vi "Relay test.vi"() -> ()   [LabVIEW 2021]
uses:
  enums/main_prog_state.ctl
  enums/init_state.ctl
  Master CR.lvclass
  Param/TCP Param/TCP Param.lvclass
  D:/my_projects/projects/Algorithms/Labview/21/Master CR/Param/Param.lvclass
  Master CR.lvclass/Master CR.ctl
  Param/Param.lvclass/Param.ctl
  Param/TCP Param/TCP Param.lvclass/TCP Param.ctl
  <vilib>/Platform/TimedLoop/XDataNode/timing_clust.ctl
  <vilib>/Platform/TimedLoop/XDataNode/nitl_modes.ctl
  <vilib>/Platform/TimedLoop/XDataNode/wakeup.ctl
  enums/close_state.ctl
  Data/Data Model/Read Data Model.vi
  <vilib>/Utility/config.llb/Read Key (String).vi
  <vilib>/Utility/config.llb/Write Key (String).vi
  <vilib>/Platform/TimedLoop/XDataNode/XDataNode.xnode
  Modbus_v121c/Data Model/Device Data Model.lvclass
  <vilib>/Platform/TimedLoop/XDataNode/XDNodeRunTimeDep.lvlib
  enums/Param_MB test.lvlib
  Param/Param.lvclass
  <vilib>/Utility/config.llb/NI_LVConfig.lvlib
panel:
  out "N2":u64
  out "N1":u64
  in  "Write":bool
  in  "Read":bool
  out "connects":bool[](array[boolean])
  out "DI":bool[](array[boolean])
  in  "DO":bool[](array[boolean])
  in  "AOint":u16[](array[numeric])
  out "comm error":errorcluster
  out "initialise error":errorcluster
  in  "EP_on":bool
  in  "tick":i64=250 caption="Время цикла основной программы" min=5 max=1000 step=1
  in  "stop":bool
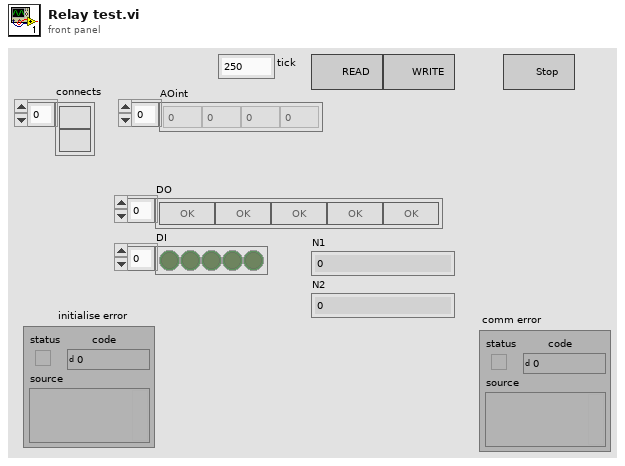
[diagram p1: front panel]
types:
  T1 = cluster{"conn_timeout":i32, "reconn_timeout":i32, "N attempt max":i32, "t_reset_TTL":i32, "write_timeout":i32, "read_timeout":i32, "period":i32}[]
  T2 = cluster{"Remote IP Address":string, "Remote Port":u16}[]
  T3 = typedef "Param_MB test.lvlib/init_state.ctl" = enum16{"Init Data", "Init TMPs", "Init system DB", "Init data DB", "Read Enums", "Init arrays", "Init KFM", "Init Param", "Init AI param", "Init DI param", "Init AO param", "Init DO param", "Init ALR param", "Init save progs", "Read OPC param", "Init Shared Variables", "Init regulators", "Init heaters", "Init Y defs", "Exit"}
  T4 = typedef "Param_MB test.lvlib/main_prog_state.ctl" = enum16{"Read_AI_Param", "Read_DI_Param", "Read_AO_Param", "Read_DO_Param", "Read_ALR_ON_OFF", "Read_ALR_Param", "Read_Param", "Read_REG_Param", "Timers", "AI", "DI", "SendAItoScada", "SendDItoScada", "Alarms", "SendAItoDB", "SendDItoDB", "SendALRtoDB", "Messages", "Controls", "Control HT1", "QN_control", "QN", "QN_state", "Control EB3", "Outputs", "Exit"}
  T5 = cluster{"KFM":string[], "PAR":string[], "AI":string[], "DI":string[], "DI_fast":string[], "AO":string[], "Regs":string[], "DO":string[], "ALR":string[], "System":string[]}
  T6 = typedef "NI_LVConfig.lvlib/Config Data RefNum.ctl" = refnum<k1>
  T7 = cluster{"Enums":cluster{"KFM":string[], "PAR":string[], "AI":string[], "DI":string[], "DI_fast":string[], "AO":string[], "Regs":string[], "DO":string[], "ALR":string[], "System":string[]}, "MBs":refnum<class "Master CR.lvclass">[], "N":string[]}
  T8 = cluster{"current time":timestamp, "Timer_1s":bool, "Timer_10s":bool, "Timer_1day":bool}
  T9 = typedef "XDNodeRunTimeDep.lvlib/timing_clust.ctl" = cluster{"Expected End [f-1]":u64, "Actual End [f-1]":u64, "Finished Late? [f-1]":bool, "Expected End [i-1]":u64, "Actual End [i-1]":u64, "Finished Late? [i-1]":bool, "Expected Start [i]":u64, "Actual Start [i]":u64, "Expected Start [f]":u64, "Actual Start [f]":u64, "Source Name":string, "Structure Name":string, "Period":i64, "Deadline":i64, "Offset":i64, "Start":i64, "Priority":i32, "Timeout":i32, "Mode":T10, "Wakeup Reason":T11, "Error":errorcluster, "Source Type":string, "Secondary Source Type":string, "Global End Time":u64, "Global Start Time":u64, "Frame Duration":u64, "Iteration Duration":u64, "Assigned CPU":i32, "I/O Scan Engine Mode":u32}
  T10 = typedef "XDNodeRunTimeDep.lvlib/nitl_modes.ctl" = enum32{"No Change", "Process missed periods, maintain original phase", "Discard missed periods, maintain original phase", "Process missed periods, ignore original phase", "Discard missed periods, ignore original phase"}
  T11 = typedef "XDNodeRunTimeDep.lvlib/wakeup.ctl" = enum32{"Normal", "Aborted", "Asynchronous wakeup", "Timing source error", "Timed loop error", "Timeout"}
  T12 = typedef "Param_MB test.lvlib/close_state.ctl" = enum16{"QN_state notifier", "QN_control_queue", "ALR notifires", "ALR", "DO notifires", "DO", "AO notifires", "AO", "DI notifres", "DI", "AI notifires", "AI", "OPC", "Param", "SaveMessageProg", "KFM DadaRef", "KFM Registers", "KFM StatusRef", "Exit"}
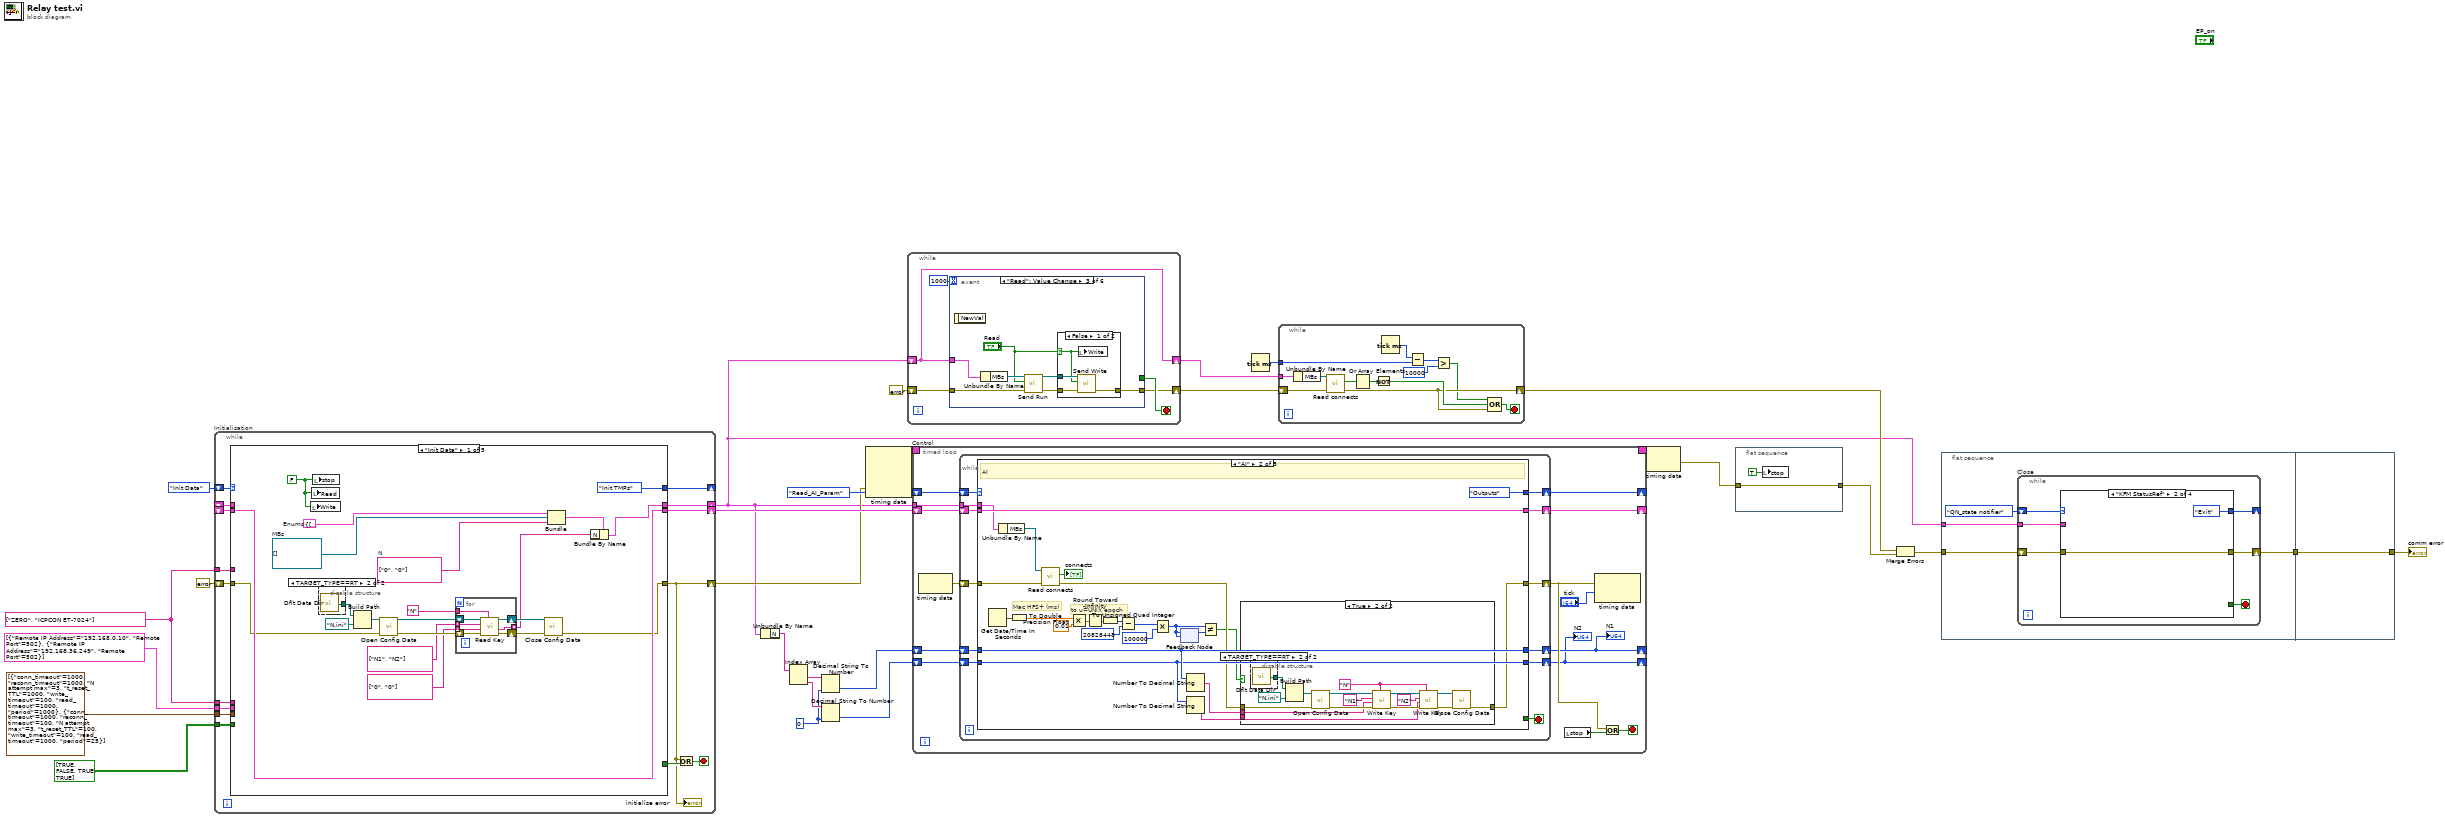
[diagram p0: block diagram]
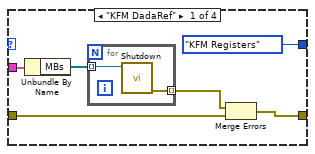
[diagram p2: hidden frame]
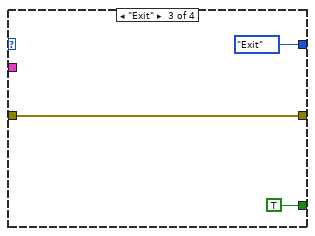
[diagram p3: hidden frame]
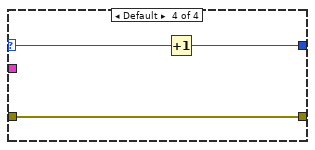
[diagram p4: hidden frame]
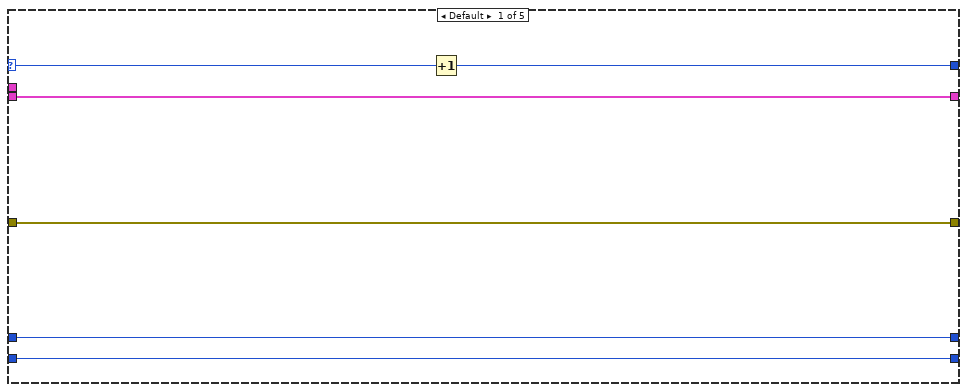
[diagram p5: hidden frame]
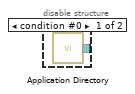
[diagram p7: hidden frame]
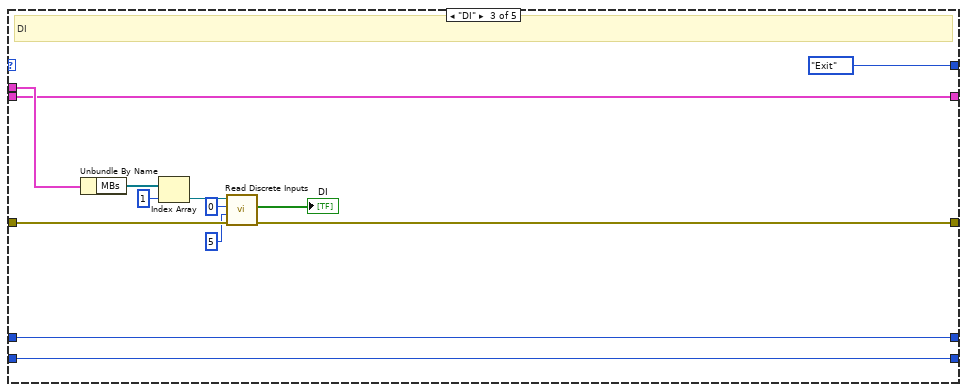
[diagram p8: hidden frame]
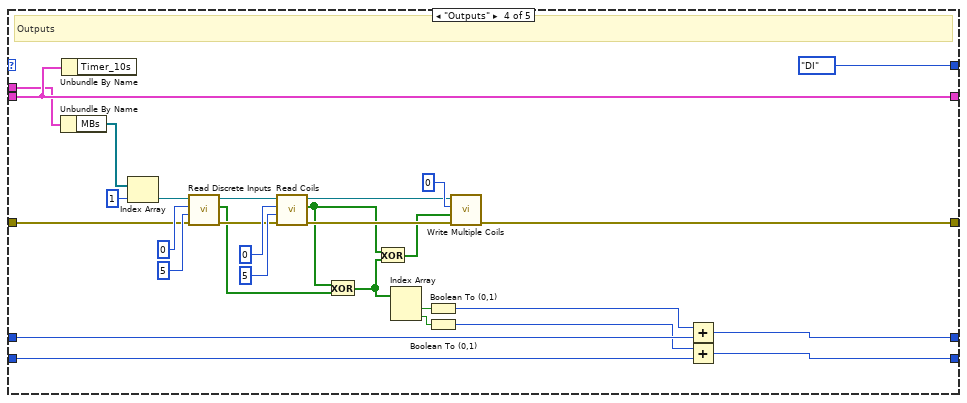
[diagram p9: hidden frame]
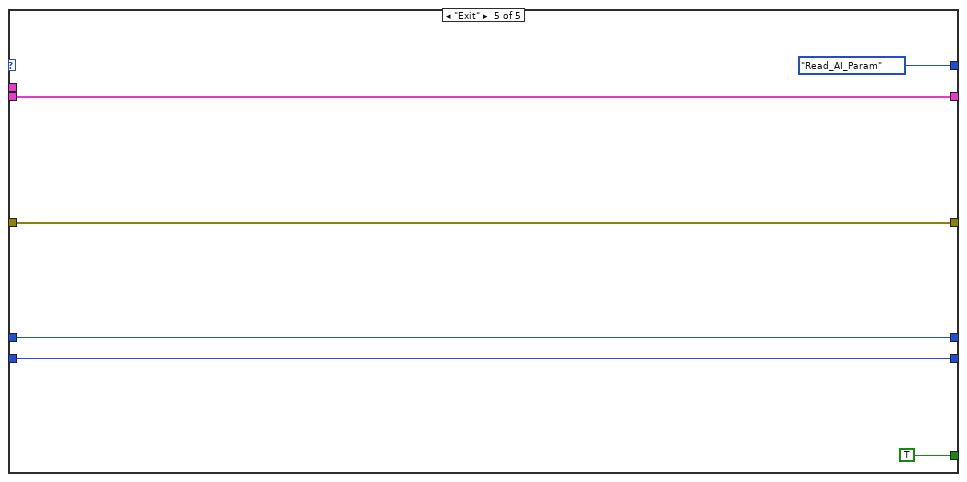
[diagram p10: hidden frame]
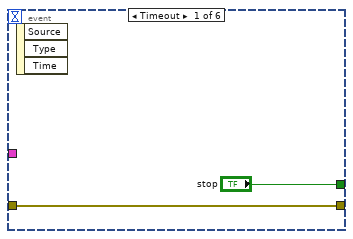
[diagram p11: hidden frame]
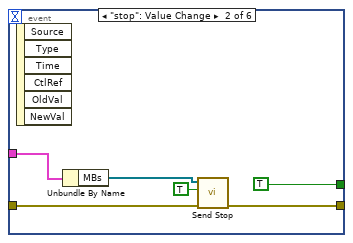
[diagram p12: hidden frame]
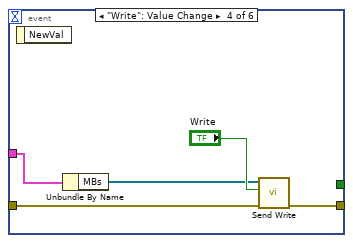
[diagram p14: hidden frame]
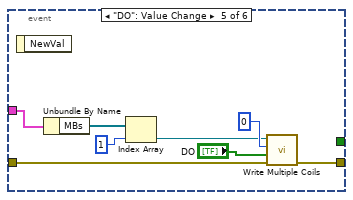
[diagram p15: hidden frame]
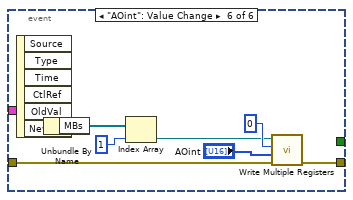
[diagram p16: hidden frame]
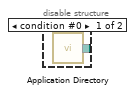
[diagram p17: hidden frame]
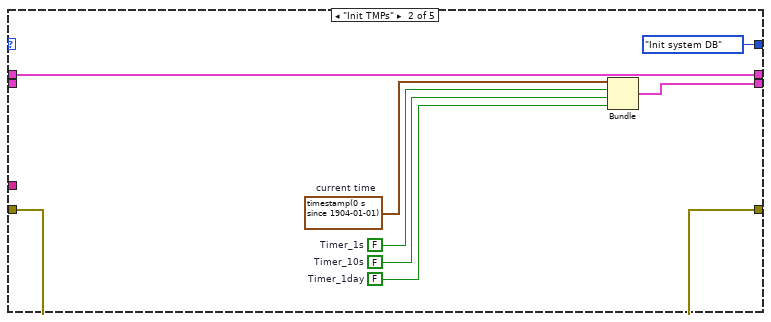
[diagram p18: hidden frame]
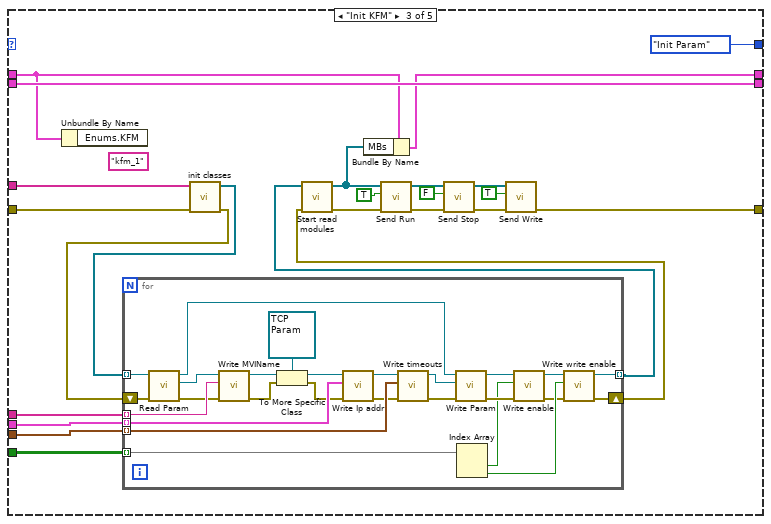
[diagram p19: hidden frame]
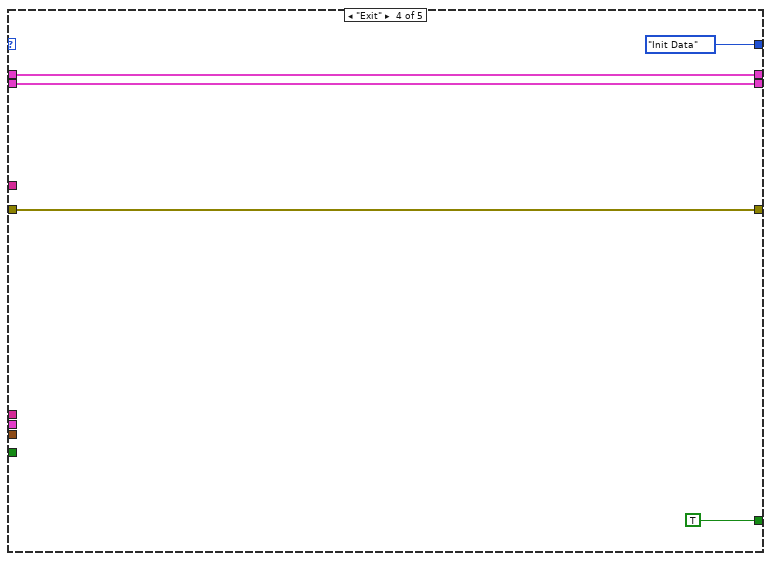
[diagram p20: hidden frame]
diagram:
  w3 = u64 0
  w15 = string[] ["ZERO", "ICPCON ET-7024"] ("MVIName")
  n1 = while "Initialisation" {
    shift-right: [w34] -> w14
    shift-left: errorcluster {"status"=FALSE, "code"=0, "source"=""} ("error out") -> [w40]
    shift-right: [w43] -> w7
    shift-left: _ -> [w41]
    shift-right: [w39] -> _
    shift-left: init_state."Init Data" -> [w42]
    shift-right: [w36] -> w22
    shift-left: _ -> [w35]
    tunnel: w15 -> [w33]
    tunnel: T2 [{"Remote IP Address"="192.168.0.10", "Remote Port"=502}, {"Remote IP Address"="192.168.36.249", "Remote Port"=502}] ("IP Address") -> [w32]
    tunnel: T1 [{"conn_timeout"=1000, "reconn_timeout"=1000, "N attempt max"=3, "t_reset_TTL"=1000, "write_timeout"=100, "read_timeout"=1000, "period"=1000}, {"conn_timeout"=1000, "reconn_timeout"=100, "N attempt max"=3, "t_reset_TTL"=100, "write_timeout"=100, "read_timeout"=1000, "period"=25}] ("timeouts") -> [w31]
    tunnel: bool[][] [[TRUE, FALSE], [TRUE, TRUE]] ("enable") -> [w30]
    tunnel: w15 -> [w29]
    stop <- w37 stop-if-true
    # "Initialisation"
    n2 = case shown="\"Init Data\"" w42 {
      tunnel: [w49 w81 w85 w135 w138] -> w34
      selector: w42 -> [_ _ _ _ w141]
      tunnel: [w44 w80 w87 w136 w139] -> w43
      tunnel: w41 -> [_ w80 w104 w136 w139]
      tunnel: w40 -> [w48 w81 w103 w135 w138]
      tunnel: [init_state."Init TMPs" init_state."Init system DB" init_state."Init Param" init_state."Init Data" w140] -> w39
      tunnel: [_ _ _ TRUE _] -> w38
      tunnel: [w62 w79 w105 w133 w142] -> w36
      tunnel: w35 -> [w62 _ w105 w133 w142]
      tunnel: w33 -> [_ _ w98 _ _]
      tunnel: w32 -> [_ _ w97 _ _]
      tunnel: w31 -> [_ _ w96 _ _]
      tunnel: w30 -> [_ _ w95 _ _]
      tunnel: w29 -> [_ _ w94 _ _]
      frame "Init Data" {
        w47 = string[] ["0", "0"]  # N
        w60 = FALSE ("stop")
        w61 = refnum<class "Master CR.lvclass">[] []  # MBs
        w63 = T5 {"KFM"=[], "PAR"=[], "AI"=[], "DI"=[], "DI_fast"=[], "AO"=[], "Regs"=[], "DO"=[], "ALR"=[], "System"=[]}  # Enums
        n3 = local write "Write"(w60) -> ()
        n4 = local write "Read"(w60) -> ()
        n5 = local write "stop"(w60) -> ()
        n6 = disable-structure shown="TARGET_TYPE==RT" {
          disable-tunnel: [w73 w74] -> w55
          frame condition #0 {
            n7 = call <vilib>:"Application Directory.vi"() -> ("Application Directory"=w73:path)
          }
          frame condition #1 (active) {
            n8 = call <vilib>:"Dflt Data Dir.vi"() -> ("App:Default Data Directory"=w74:path)
          }
        }
        n9 = Build Path(base path=w55, name or relative path=path "N.ini" ("configuration file path")) -> (appended path=w59:path)
        n10 = call <vilib>:"Open Config Data.vi"("error in (no error)"=w48, "configuration file path"=w59) -> ("error out"=w58:errorcluster, "refnum"=w57:T6)  [unwired: 7 in, 1 out]
        n11 = for {
          tunnel: "N" ("key") -> [w69]
          shift-right: [w67] -> w53
          shift-left: w58 -> [w72]
          shift-right: [w66] -> w52
          shift-left: w57 -> [w71]
          tunnel: string[] ["N1", "N2"] -> [w70] mode=indexing
          tunnel: [w68] -> w46 mode=indexing
          tunnel: string[] ["0", "0"] -> [w65] mode=indexing
          n12 = call-poly <vilib>:"Read Key.vi"("section"=w69, "error in (no error)"=w72, "default value"=w65, "key"=w70, "refnum"=w71) -> ("error out"=w67:errorcluster, "value"=w68:string, "refnum out"=w66:T6)  [unwired: 3 in, 1 out]
        }
        n13 = call <vilib>:"Close Config Data.vi"("error in (no error)"=w53, "refnum"=w52) -> ("error out"=w49:errorcluster)  [unwired: 8 in, 1 out]
        n14 = Bundle("Enums"=w63, "MBs"=w61, "N"=w47) -> (w45:T7)  [unwired: 1 in]
        n15 = Bundle By Name(cluster=w45, "N"=w46) -> (w44:T7)
      }
      frame "Init TMPs" {
        w75 = FALSE  # Timer_10s
        w76 = FALSE  # Timer_1day
        w77 = FALSE  # Timer_1s
        w78 = timestamp(0 s since 1904-01-01)  # current time
        n16 = Bundle("current time"=w78, "Timer_1s"=w77, "Timer_10s"=w75, "Timer_1day"=w76) -> (w79:T8)  [unwired: 1 in]
      }
      frame "Init KFM" {
        (unwired) "kfm_1" ("KFMTable")
        n17 = Unbundle By Name(w104) -> ()  [unwired: 1 out]
        n18 = call "init classes.vi"("error in (no error)"=w103, "MVINames"=w94) -> ("error out"=w100:errorcluster, "MBs"=w102:refnum<class "Master CR.lvclass">[])  [unwired: 8 in]
        n19 = for {
          tunnel: w102 -> [w108] mode=indexing
          tunnel: w97 -> [w115] mode=indexing
          tunnel: w96 -> [w112] mode=indexing
          tunnel: w98 -> [w130] mode=indexing
          tunnel: w95 -> [w124] mode=indexing
          tunnel: [w120] -> w101 mode=indexing
          shift-right: [w119] -> w99
          shift-left: w100 -> [w132]
          n20 = call "Read Param.vi"("error in (no error)"=w132, "MB_TCP in"=w108) -> ("error out"=w128:errorcluster, "Param"=w107:refnum<class "Param.lvclass">, "MB_TCP out"=w127:refnum<class "Master CR.lvclass">)  [unwired: 7 in]
          n21 = call "Write MVIName.vi"("error in (no error)"=w128, "MVIName"=w130, "MB Param in"=w107) -> ("error out"=w117:errorcluster, "MB Param out"=w129:refnum<class "Param.lvclass">)  [unwired: 7 in]
          n22 = To More Specific Class(target class=refnum<class "TCP Param.lvclass"> refnum ("Param.lvlib:TCP Param.lvclass"), reference=w129, error in=w117) -> (specific class reference=w116:refnum<class "TCP Param.lvclass">, error out=w114:errorcluster)
          n23 = call "Write Ip addr.vi"("error in (no error)"=w114, "IP address"=w115, "MB Param in"=w116) -> ("error out"=w111:errorcluster, "MB Param out"=w113:refnum<class "TCP Param.lvclass">)  [unwired: 7 in]
          n24 = call "Write timeouts.vi"("error in (no error)"=w111, "timeouts"=w112, "MB Param in"=w113) -> ("error out"=w110:errorcluster, "MB Param out"=w109:refnum<class "TCP Param.lvclass">)  [unwired: 7 in]
          n25 = call "Write Param.vi"("error in (no error)"=w110, "Param"=w109, "MB_TCP in"=w127) -> ("error out"=w125:errorcluster, "MB_TCP out"=w126:refnum<class "Master CR.lvclass">)  [unwired: 7 in]
          n26 = Index Array(array=w124) -> (element #1=w123:bool, element #2=w122:bool)  [unwired: 2 in]
          n27 = call "Write enable.vi"("error in (no error)"=w125, "enable"=w123, "Master CR in"=w126) -> ("error out"=w121:errorcluster, "Master CR out"=w131:refnum<class "Master CR.lvclass">)  [unwired: 7 in]
          n28 = call "Write write enable.vi"("error in (no error)"=w121, "write enable"=w122, "Master CR in"=w131) -> ("error out"=w119:errorcluster, "Master CR out"=w120:refnum<class "Master CR.lvclass">)  [unwired: 7 in]
        }
        n29 = call "Start read modules.vi"("error in"=w99, "classes"=w101) -> ("error out"=w89:errorcluster, "classes initialised"=w88:refnum<class "Master CR.lvclass">[])  [unwired: 8 in]
        n30 = Bundle By Name(cluster=w104, "MBs"=w88) -> (w87:T7)
        n31 = call "Send Run.vi"("error in"=w89, "Run"=TRUE, "MCRs"=w88) -> ("error out"=w92:errorcluster, "MCRs out"=w93:refnum<class "Master CR.lvclass">[])  [unwired: 7 in]
        n32 = call "Send Stop.vi"("error in"=w92, "Stop"=FALSE ("Write"), "MCRs"=w93) -> ("error out"=w86:errorcluster, "MCRs out"=w84:refnum<class "Master CR.lvclass">[])  [unwired: 7 in]
        n33 = call "Send Write.vi"("error in"=w86, "Write"=TRUE, "MCRs"=w84) -> ("error out"=w85:errorcluster)  [unwired: 7 in, 1 out]
      }
      frame "Exit" {
      }
      frame Default {
        n34 = Increment(x=w141) -> (x+1=w140:T3)
      }
    }
    "initialise error" <- w34
    n35 = Or(x=w34, y=w38) -> (x .or. y?=w37:bool)
  }
  n36 = Unbundle By Name(w7) -> ("N"=w6:string[])
  n37 = Index Array(array=w6) -> (element #1=w5:string, element #2=w4:string)  [unwired: 2 in]
  n38 = Decimal String To Number(string=w5, default (0L)=w3) -> (number=w2:u64)  [unwired: 1 in, 1 out]
  n39 = Decimal String To Number(string=w4, default (0L)=w3) -> (number=w1:u64)  [unwired: 1 in, 1 out]
  n40 = node-c288(w14) -> (w28:T9)  [unwired: 3 in]
  n41 = while {
    shift-right: [w145] -> w11
    shift-left: errorcluster {"status"=FALSE, "code"=0, "source"=""} ("error out") -> [w144]
    shift-right: [w143] -> w10
    shift-left: w7 -> [w143]
    stop <- w146 stop-if-true
    n42 = event shown="[2] \"Read\": Value Change" {
      selector: _ -> [_ _ _ _ _ _]
      dyn-events: _ -> [_ _ _ _ _ _]
      timeout: 1000 -> [_ _ _ _ _ _]
      tunnel: ["stop" TRUE ("stop") _ _ _ _] -> w146
      tunnel: w143 -> [_ w150 w162 w172 w180 w188]
      tunnel: w144 -> [w148 w154 w161 w171 w177 w183]
      tunnel: [w148 w153 w156 w170 w176 w182] -> w145
      event Timeout {
        n43 = event-data() -> ()  [unwired: 1 in, 3 out]
      }
      event "stop": Value Change {
        n44 = event-data() -> ()  [unwired: 1 in, 6 out]
        n45 = Unbundle By Name(w150) -> ("MBs"=w151:refnum<class "Master CR.lvclass">[])
        n46 = call "Send Stop.vi"("error in"=w154, "Stop"=TRUE, "MCRs"=w151) -> ("error out"=w153:errorcluster)  [unwired: 7 in, 1 out]
      }
      event "Read": Value Change {
        n47 = event-data() -> ()  [unwired: 1 in, 1 out]
        n48 = Unbundle By Name(w162) -> ("MBs"=w160:refnum<class "Master CR.lvclass">[])
        n49 = call "Send Run.vi"("error in"=w161, "Run"="Read", "MCRs"=w160) -> ("error out"=w158:errorcluster, "MCRs out"=w157:refnum<class "Master CR.lvclass">[])  [unwired: 7 in]
        n50 = case shown="False" "Read" {
          selector: "Read" -> [w164 _]
          tunnel: w158 -> [w166 w167]
          tunnel: w157 -> [w165 _]
          tunnel: [w163 w167] -> w156
          frame False {
            n51 = call "Send Write.vi"("error in"=w166, "Write"=w164, "MCRs"=w165) -> ("error out"=w163:errorcluster)  [unwired: 7 in, 1 out]
            n52 = local write "Write"(w164) -> ()
          }
          frame True {
          }
        }
      }
      event "Write": Value Change {
        n53 = event-data() -> ()  [unwired: 1 in, 1 out]
        n54 = Unbundle By Name(w172) -> ("MBs"=w168:refnum<class "Master CR.lvclass">[])
        n55 = call "Send Write.vi"("error in"=w171, "Write"="Write", "MCRs"=w168) -> ("error out"=w170:errorcluster)  [unwired: 7 in, 1 out]
      }
      event "DO": Value Change {
        n56 = event-data() -> ()  [unwired: 1 in, 1 out]
        n57 = Unbundle By Name(w180) -> ("MBs"=w174:refnum<class "Master CR.lvclass">[])
        n58 = Index Array(array=w174, index=1) -> (element=w173:refnum<class "Master CR.lvclass">)
        n59 = call-dynamic "Write Multiple Coils.vi"("error in"=w177, "coils"="DO", "starting address"=u16 0, "Master CR in"=w173) -> ("error out"=w176:errorcluster)  [unwired: 6 in, 1 out]
      }
      event "AOint": Value Change {
        n60 = event-data() -> ()  [unwired: 1 in, 6 out]
        n61 = Unbundle By Name(w188) -> ("MBs"=w186:refnum<class "Master CR.lvclass">[])
        n62 = Index Array(array=w186, index=1) -> (element=w181:refnum<class "Master CR.lvclass">)
        n63 = call-dynamic "Write Multiple Registers.vi"("error in"=w183, "register values"="AOint", "starting address"=u16 0, "Master CR in"=w181) -> ("error out"=w182:errorcluster)  [unwired: 6 in, 1 out]
      }
    }
  }
  n64 = timed-loop "Control" {
    tunnel: w7 -> [w202]
    shift-right: [w200] -> _
    shift-left: w22 -> [w201]
    timing: w28 -> [_]
    timing-out: [_] -> w27
    shift-right: [w198] -> _
    shift-left: main_prog_state."Read_AI_Param" -> [w197]
    shift-right: [w192] -> _
    shift-left: w2 -> [w191]
    shift-right: [w189] -> _
    shift-left: w1 -> [w190]
    stop <- w195 stop-if-true
    n65 = node-c288() -> (w199:errorcluster)  [unwired: 1 in]
    n66 = while {
      tunnel: w202 -> [w214]
      shift-right: [w212] -> w200
      shift-left: w201 -> [w213]
      shift-right: [w207] -> w193
      shift-left: w199 -> [w211]
      shift-right: [w210] -> w198
      shift-left: w197 -> [w209]
      shift-right: [w206] -> w192
      shift-left: w191 -> [w204]
      shift-right: [w205] -> w189
      shift-left: w190 -> [w203]
      stop <- w208 stop-if-true
      n67 = case shown="\"AI\"" w209 {
        tunnel: w211 -> [w217 w243 w273 w294 w308]
        tunnel: w214 -> [_ w240 w275 w303 _]
        tunnel: w213 -> [w219 w242 w274 w304 w309]
        tunnel: [w219 w242 w274 w304 w309] -> w212
        selector: w209 -> [w220 _ _ _ _]
        tunnel: [w218 main_prog_state."Outputs" main_prog_state."Exit" main_prog_state."DI" main_prog_state."Read_AI_Param"] -> w210
        tunnel: [_ _ _ _ TRUE] -> w208
        tunnel: [w217 w224 w271 w302 w308] -> w207
        tunnel: [w216 w227 w265 w282 w307] -> w206
        tunnel: [w215 w226 w264 w279 w306] -> w205
        tunnel: w204 -> [w216 w227 w265 w281 w307]
        tunnel: w203 -> [w215 w226 w264 w280 w306]
        frame Default {
          n68 = Increment(x=w220) -> (x+1=w218:T4)
        }
        frame "AI" {
          # "to u=UNIX epoch"
          # "Mac HFS+ (ms)"
          # "AI"
          n69 = Get Date/Time In Seconds() -> (seconds since 1Jan1904=w238:timestamp)
          n70 = Unbundle By Name(w240) -> ("MBs"=w239:refnum<class "Master CR.lvclass">[])
          n71 = To Double Precision Float(number=w238) -> (double precision float=w228:dbl)
          n72 = call "Read connects.vi"("error in (no error)"=w243, "MCRs in"=w239) -> ("error out"=w225:errorcluster, "connects"=→"connects":bool[])  [unwired: 7 in, 1 out]
          n73 = Multiply(x=w228, y=0.01) -> (x*y=w230:dbl)
          n74 = Round Toward -Infinity(1:w230) -> (0:w229:dbl)
          n75 = To Unsigned Quad Integer(1:w229) -> (0:w232:u64)
          n76 = Subtract(x=w232, y=u64 20828448) -> (x-y=w231:u64)
          n77 = Multiply(x=w231, y=u64 100000) -> (x*y=w237:u64)
          n78 = feedback #1(w237) -> (w236:u64)
          n79 = feedback-in #1(w237) -> ()
          n80 = Number To Decimal String(number=w227) -> (decimal integer string=w223:string)  [unwired: 1 in]
          n81 = Number To Decimal String(number=w226) -> (decimal integer string=w222:string)  [unwired: 1 in]
          n82 = Not Equal?(x=w237, y=w236) -> (x != y?=w221:bool)
          n83 = case shown="True" w221 {
            tunnel: w225 -> [w245 w250]
            tunnel: [w245 w249] -> w224
            tunnel: w223 -> [_ w248]
            tunnel: w222 -> [_ w247]
            frame False {
            }
            frame True {
              w246 = "N" ("key")
              n84 = disable-structure shown="TARGET_TYPE==RT" {
                disable-tunnel: [w262 w263] -> w254
                frame condition #0 {
                  n85 = call <vilib>:"Application Directory.vi"() -> ("Application Directory"=w262:path)
                }
                frame condition #1 (active) {
                  n86 = call <vilib>:"Dflt Data Dir.vi"() -> ("App:Default Data Directory"=w263:path)
                }
              }
              n87 = Build Path(base path=w254, name or relative path=path "N.ini" ("configuration file path")) -> (appended path=w251:path)
              n88 = call <vilib>:"Open Config Data.vi"("error in (no error)"=w250, "configuration file path"=w251) -> ("error out"=w252:errorcluster, "refnum"=w253:T6)  [unwired: 7 in, 1 out]
              n89 = call-poly <vilib>:"Write Key.vi"("section"=w246, "error in (no error)"=w252, "value"=w248, "key"="N1", "refnum"=w253) -> ("error out"=w257:errorcluster, "refnum out"=w256:T6)  [unwired: 4 in, 1 out]
              n90 = call-poly <vilib>:"Write Key.vi"("section"=w246, "error in (no error)"=w257, "value"=w247, "key"="N2", "refnum"=w256) -> ("error out"=w261:errorcluster, "refnum out"=w260:T6)  [unwired: 4 in, 1 out]
              n91 = call <vilib>:"Close Config Data.vi"("error in (no error)"=w261, "refnum"=w260) -> ("error out"=w249:errorcluster)  [unwired: 8 in, 1 out]
            }
          }
        }
        frame "DI" {
          # "DI"
          n92 = Unbundle By Name(w275) -> ("MBs"=w270:refnum<class "Master CR.lvclass">[])
          n93 = Index Array(array=w270, index=1) -> (element=w267:refnum<class "Master CR.lvclass">)
          n94 = call "Read Discrete Inputs.vi"("error in"=w273, "number of inputs"=u16 5 ("number of coils"), "starting address"=u16 0, "Master CR in"=w267) -> ("error out"=w271:errorcluster, "discrete inputs"=→"DI":bool[])  [unwired: 5 in, 1 out]
        }
        frame "Outputs" {
          # "Outputs"
          n95 = Unbundle By Name(w303) -> ("MBs"=w300:refnum<class "Master CR.lvclass">[])
          n96 = Unbundle By Name(w304) -> ()  [unwired: 1 out]
          n97 = Index Array(array=w300, index=1) -> (element=w293:refnum<class "Master CR.lvclass">)
          n98 = call "Read Discrete Inputs.vi"("error in"=w294, "number of inputs"=u16 5, "starting address"=u16 0, "Master CR in"=w293) -> ("error out"=w292:errorcluster, "discrete inputs"=w290:bool[], "Master CR out"=w291:refnum<class "Master CR.lvclass">)  [unwired: 5 in]
          n99 = call "Read Coils.vi"("error in"=w292, "number of inputs"=u16 5, "starting address"=u16 0, "Master CR in"=w291) -> ("error out"=w289:errorcluster, "coils"=w286:bool[], "Master CR out"=w288:refnum<class "Master CR.lvclass">)  [unwired: 5 in]
          n100 = Exclusive Or(1:w290, 2:w286) -> (0:w285:bool[])
          n101 = Exclusive Or(1:w285, 2:w286) -> (0:w287:bool[])
          n102 = Index Array(array=w285) -> (element #1=w284:bool, element #2=w283:bool)  [unwired: 2 in]
          n103 = Boolean To (0,1)(Boolean=w284) -> (0, 1=w278:i16)
          n104 = Boolean To (0,1)(Boolean=w283) -> (0, 1=w277:i16)
          n105 = call-dynamic "Write Multiple Coils.vi"("error in"=w289, "coils"=w287, "starting address"=u16 0, "Master CR in"=w288) -> ("error out"=w302:errorcluster)  [unwired: 6 in, 1 out]
          n106 = Add(x=w278, y=w281) -> (x+y=w282:u64)
          n107 = Add(x=w277, y=w280) -> (x+y=w279:u64)
        }
        frame "Exit" {
        }
      }
    }
    "N1" <- w192
    "N2" <- w189
    n108 = local read "stop"() -> (w194:bool)
    n109 = node-c288(w193, "tick") -> ()  [unwired: 1 out]
    n110 = Or(x=w193, y=w194) -> (x .or. y?=w195:bool)
  }
  n111 = Tick Count (ms)() -> (millisecond timer value=w9:u32)
  n112 = while {
    shift-right: [w323] -> w8
    shift-left: w11 -> [w330]
    tunnel: w10 -> [w327]
    tunnel: w9 -> [w321]
    stop <- w325 stop-if-true
    n113 = Unbundle By Name(w327) -> ("MBs"=w326:refnum<class "Master CR.lvclass">[])
    n114 = call "Read connects.vi"("error in (no error)"=w330, "MCRs in"=w326) -> ("error out"=w323:errorcluster, "connects"=w329:bool[])  [unwired: 7 in, 1 out]
    n115 = Or Array Elements(Boolean array=w329) -> (logical OR=w328:bool)
    n116 = Not(x=w328) -> (.not. x?=w324:bool)
    n117 = Tick Count (ms)() -> (millisecond timer value=w322:u32)
    n118 = Subtract(x=w322, y=w321) -> (x-y=w320:u32)
    n119 = Greater?(x=w320, y=u32 10000) -> (0:w318:bool)
    n120 = Compound Arithmetic op=OR(w318, w324, w323) -> (w325:bool)
  }
  n121 = node-c288(w27) -> (w13:errorcluster)
  n122 = flat-sequence {
    tunnel: [w331] -> w12
    tunnel: w13 -> [w331]
    frame #0 {
      n123 = local write "stop"(TRUE ("stop")) -> ()
    }
  }
  n124 = Merge Errors(w8, w12) -> (w21:errorcluster)
  n125 = flat-sequence {
    tunnel: w7 -> [w335]
    tunnel: w21 -> [w334]
    tunnel: [w333] -> w20
    tunnel: [w359] -> w25
    tunnel: w20 -> [w359]
    frame #0 {
      n126 = while "Close" {
        shift-right: [w341] -> _
        shift-left: close_state."QN_state notifier" ("Init_state") -> [w342]
        tunnel: w335 -> [w339]
        shift-right: [w337] -> w333
        shift-left: w334 -> [w338]
        stop <- w340 stop-if-true
        n127 = case shown="\"KFM StatusRef\"" w342 {
          selector: w342 -> [_ _ _ w358]
          tunnel: [close_state."KFM Registers" close_state."Exit" close_state."Exit" w357] -> w341
          tunnel: [_ _ TRUE _] -> w340
          tunnel: w339 -> [w348 _ _ _]
          tunnel: w338 -> [w346 w351 w354 w356]
          tunnel: [w345 w351 w354 w356] -> w337
          frame "KFM DadaRef" {
            n128 = Unbundle By Name(w348) -> ("MBs"=w344:refnum<class "Master CR.lvclass">[])
            n129 = for {
              tunnel: w344 -> [w350] mode=indexing
              tunnel: [w349] -> w343 mode=indexing
              n130 = call-dynamic "Shutdown.vi"("MB in"=w350) -> ("error out"=w349:errorcluster)  [unwired: 10 in]
            }
            n131 = Merge Errors(w343, w346) -> (w345:errorcluster)
          }
          frame "KFM StatusRef" {
          }
          frame "Exit" {
          }
          frame Default {
            n132 = Increment(x=w358) -> (x+1=w357:T12)
          }
        }
      }
    }
    frame #1 {
    }
  }
  "comm error" <- w25
